vi "Initialize Numeric Tab.vi"(8 "error in (no error)":errorcluster, 11 "Numeric Data Type in":refnum<class "Numeric Data Type.lvclass">) -> (0 "error out":errorcluster, 3 "Numeric Data Type (dub)":refnum<class "Numeric Data Type.lvclass">)   [LabVIEW 2018, in "Numeric Data Type.lvclass"]
uses:
  Numeric Data Type.lvclass
  Precision Type.ctl
  Numeric Data Type.lvclass/Numeric Data Type.ctl
  Reference Digits.vi
  Reference Precision Type.vi
  Reference Hide Zeros.vi
  Reference Exponent.vi
  Reference Min Field Width.vi
  Reference Use Min Width.vi
  Reference Padding.vi
  Reference Display Type.vi
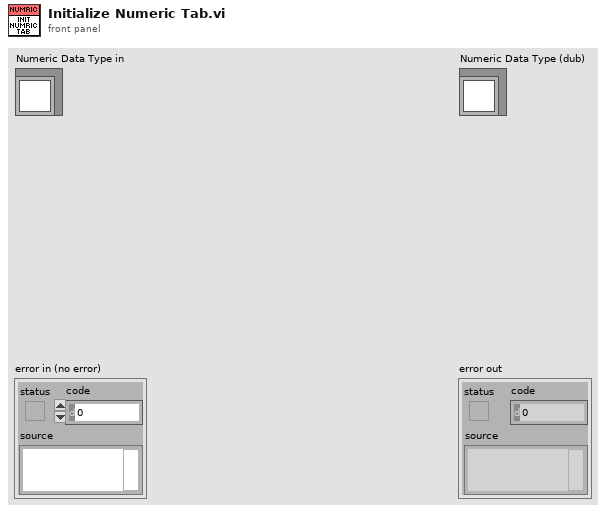
[diagram p1: front panel]
types:
  T1 = enum8{"Enabled", "Disabled", "Disabled and Grayed Out"}
  T2 = typedef "Numeric Data Type.lvclass/Precision Type.ctl" = enum16{"Digits of precision", "Significant digits"}
  T3 = typedef "Numeric Data Type.lvclass/Numeric Info.ctl" = cluster{"Minimum Field Width":i32, "Digits of Precision":i32, "Numeric Format":T4, "Precision Type":T2, "Hide trailing zeros":bool, "exponent":bool, "just/pad":T5, "Modifiers":string}
  T4 = typedef "Numeric Data Type.lvclass/Numeric Format Enum.ctl" = enum16{"Floating Point Notation", "Scientific Notation", "Engineering Notation", "SI Notation", "<not used>", "Decimal", "Hexadecimal", "Octal", "Binary", "<not used 2>", "Absolute Time", "Relative Time"}
  T5 = typedef "Numeric Data Type.lvclass/Padding.ctl" = enum16{"Pad with spaces on left", "Pad with spaces on right", "Pad with zeros on left"}
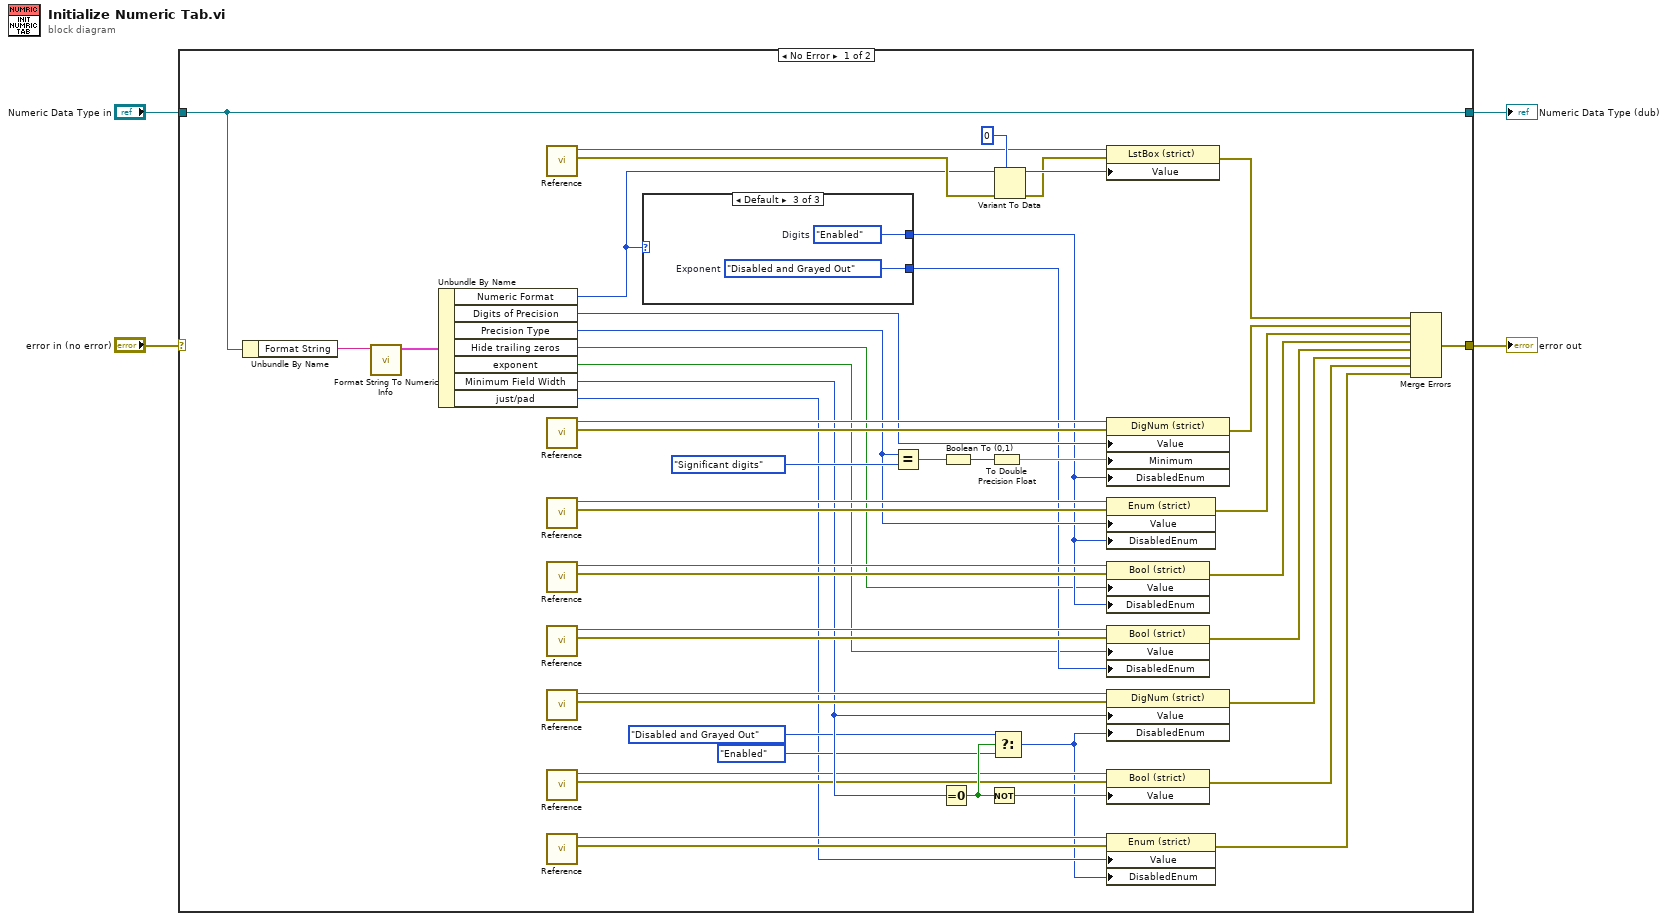
[diagram p0: block diagram]
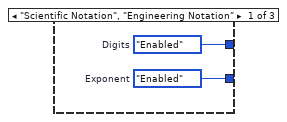
[diagram p2: hidden frame]
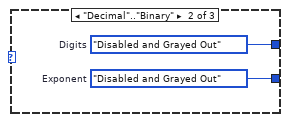
[diagram p3: hidden frame]
diagram:
  n1 = case shown="No Error" "error in (no error)" {
    selector: "error in (no error)" -> [_ w61]
    tunnel: [w16 w61] -> w3
    tunnel: [w53 w60] -> w1
    tunnel: "Numeric Data Type in" -> [w53 w60]
    frame No Error {
      n2 = Unbundle By Name(w53) -> ("Format String"=w52:string)
      n3 = call "Format String To Numeric Info.vi"("Format String"=w52) -> ("Numeric Format & Precision Info"=w51:T3)  [unwired: 10 in]
      n4 = Unbundle By Name(w51) -> ("Numeric Format"=w6:T4, "Digits of Precision"=w44:i32, "Precision Type"=w41:T2, "Hide trailing zeros"=w37:bool, "exponent"=w33:bool, "Minimum Field Width"=w30:i32, "just/pad"=w21:T5)
      n5 = call-poly "Reference.vi"() -> ("error out"=w8:errorcluster, "Display Type"=w17:refnum<vi>)  [unwired: 10 in]
      n6 = call-poly "Reference.vi"() -> ("error out"=w49:errorcluster, "Digits"=w50:refnum<vi>)  [unwired: 10 in]
      n7 = call-poly "Reference.vi"() -> ("error out"=w42:errorcluster, "Precision Type"=w43:refnum<vi>)  [unwired: 10 in]
      n8 = call-poly "Reference.vi"() -> ("error out"=w40:errorcluster, "Hide Zeros"=w39:refnum<vi>)  [unwired: 10 in]
      n9 = call-poly "Reference.vi"() -> ("error out"=w35:errorcluster, "Exponent"=w36:refnum<vi>)  [unwired: 10 in]
      n10 = call-poly "Reference.vi"() -> ("error out"=w32:errorcluster, "Min Field Width"=w31:refnum<vi>)  [unwired: 10 in]
      n11 = call-poly "Reference.vi"() -> ("error out"=w25:errorcluster, "Use Min Width"=w26:refnum<vi>)  [unwired: 10 in]
      n12 = call-poly "Reference.vi"() -> ("error out"=w23:errorcluster, "Padding"=w22:refnum<vi>)  [unwired: 10 in]
      n13 = case shown="Default" w6 {
        tunnel: [w54 w57 w58] -> w34
        tunnel: [w55 w56 w59] -> w38
        frame "Scientific Notation", "Engineering Notation" {
          w55 = T1."Enabled"  # Digits
          w54 = T1."Enabled"  # Exponent
        }
        frame "Decimal".."Binary" {
          w56 = T1."Disabled and Grayed Out"  # Digits
          w57 = T1."Disabled and Grayed Out"  # Exponent
        }
        frame Default {
          w59 = T1."Enabled"  # Digits
          w58 = T1."Disabled and Grayed Out"  # Exponent
        }
      }
      n14 = Equal?(x=w41, y=Precision_Type."Significant digits" ("Precision Type")) -> (x = y?=w47:bool)
      n15 = Equal To 0?(x=w30) -> (x = 0?=w29:bool)
      n16 = Boolean To (0,1)(Boolean=w47) -> (0, 1=w46:i16)
      n17 = Not(x=w29) -> (.not. x?=w24:bool)
      n18 = To Double Precision Float(number=w46) -> (double precision float=w45:dbl)
      n19 = Select(t=T1."Disabled and Grayed Out", s=w29, f=T1."Enabled") -> (s? t:f=w20:T1)
      n20 = Variant To Data(error in=w8, type=0, Variant=w6) -> (data=w18:i32, error out=w7:errorcluster)
      n21 = property class="LstBox (strict)"(reference=w17, error in=w7, "Value"=w18) -> (error out=w5:errorcluster)  [unwired: 1 out]
      n22 = property class="DigNum (strict)"(reference=w50, error in=w49, "Value"=w44, "Minimum"=w45, "DisabledEnum"=w38) -> (error out=w15:errorcluster)  [unwired: 1 out]
      n23 = property class="Enum (strict)"(reference=w43, error in=w42, "Value"=w41, "DisabledEnum"=w38) -> (error out=w14:errorcluster)  [unwired: 1 out]
      n24 = property class="Bool (strict)"(reference=w39, error in=w40, "Value"=w37, "DisabledEnum"=w38) -> (error out=w13:errorcluster)  [unwired: 1 out]
      n25 = property class="Bool (strict)"(reference=w36, error in=w35, "Value"=w33, "DisabledEnum"=w34) -> (error out=w12:errorcluster)  [unwired: 1 out]
      n26 = property class="DigNum (strict)"(reference=w31, error in=w32, "Value"=w30, "DisabledEnum"=w20) -> (error out=w11:errorcluster)  [unwired: 1 out]
      n27 = property class="Bool (strict)"(reference=w26, error in=w25, "Value"=w24) -> (error out=w10:errorcluster)  [unwired: 1 out]
      n28 = property class="Enum (strict)"(reference=w22, error in=w23, "Value"=w21, "DisabledEnum"=w20) -> (error out=w9:errorcluster)  [unwired: 1 out]
      n29 = Merge Errors(w5, w15, w14, w13, w12, w11, w10, w9) -> (w16:errorcluster)
    }
    frame Error {
    }
  }
  "error out" <- w3
  "Numeric Data Type (dub)" <- w1
